vi "Project Root Path.vi"() -> (2 "stripped path":path)   [LabVIEW 2018]
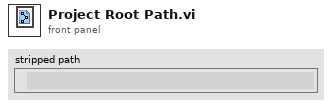
[diagram p1: front panel]
types:
  T1 = enum32{"invalid app kind", "Development System", "Run Time System", "Student Edition", "Embedded LabVIEW", "Evaluation", "Custom"}
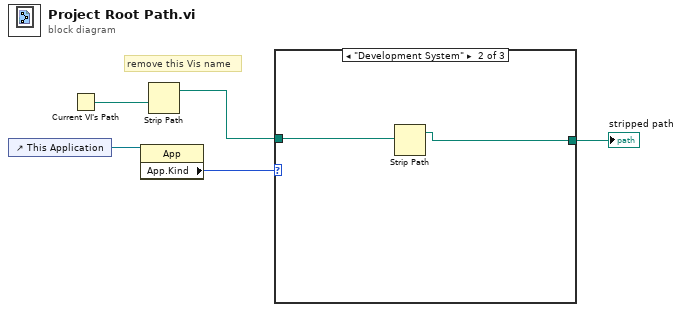
[diagram p0: block diagram]
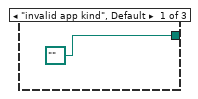
[diagram p2: hidden frame]
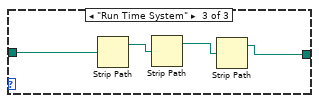
[diagram p3: hidden frame]
diagram:
  # "remove this Vis name"
  n1 = control-ref of="This Application"() -> (w5:refnum<vi>)
  n2 = Current VI's Path() -> (path=w3:path)
  n3 = property class="App"(reference=w5) -> ("App.Kind"=w4:T1)  [unwired: 1 in, 2 out]
  n4 = Strip Path(path=w3) -> (stripped path=w1:path)  [unwired: 1 out]
  n5 = case shown="\"Development System\"" w4 {
    tunnel: w1 -> [_ w7 w9]
    tunnel: [path "" ("stripped path") w8 w10] -> w2
    frame "invalid app kind", Default {
    }
    frame "Development System" {
      n6 = Strip Path(path=w7) -> (stripped path=w8:path)  [unwired: 1 out]
    }
    frame "Run Time System" {
      n7 = Strip Path(path=w9) -> (stripped path=w11:path)  [unwired: 1 out]
      n8 = Strip Path(path=w11) -> (stripped path=w12:path)  [unwired: 1 out]
      n9 = Strip Path(path=w12) -> (stripped path=w10:path)  [unwired: 1 out]
    }
  }
  "stripped path" <- w2
